vi "数据平滑.vi"(8 "Reference data in":cluster{"参考数值":dbl[], "参考数值时间戳":timestamp[]}, 10 "Para":T2 {"切换阈值" format="%#_6f"}, 11 "data in":cluster{"数值":dbl, "时间标识":timestamp}) -> (0 "Reference data out":cluster{"参考数值":dbl[], "参考数值时间戳":timestamp[]}, 3 "data out":T1)   [LabVIEW 2016, in "仿真数据.lvlib"]
uses:
  <vilib>/Analysis/NI_AALBase.lvlib
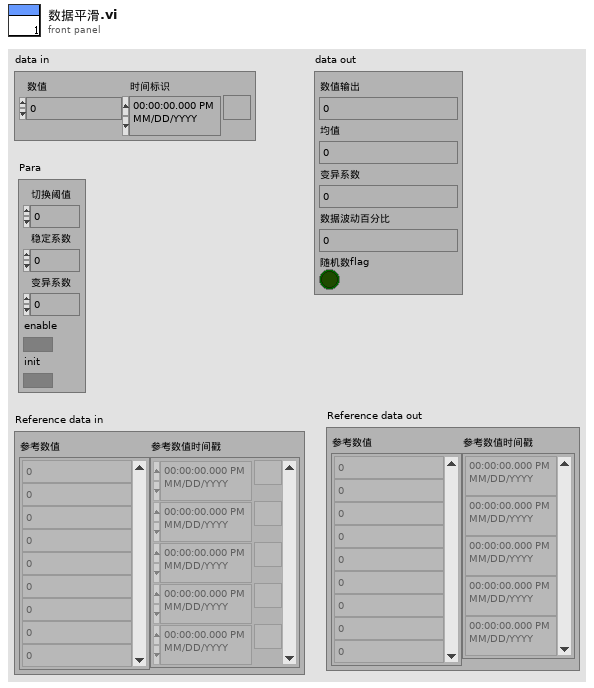
[diagram p1: front panel]
types:
  T1 = cluster{"数值输出":dbl, "均值":dbl, "变异系数":dbl, "数据波动百分比":dbl, "随机数flag":bool}
  T2 = cluster{"切换阈值":dbl, "稳定系数":dbl, "变异系数":dbl, "enable":bool, "init":bool}
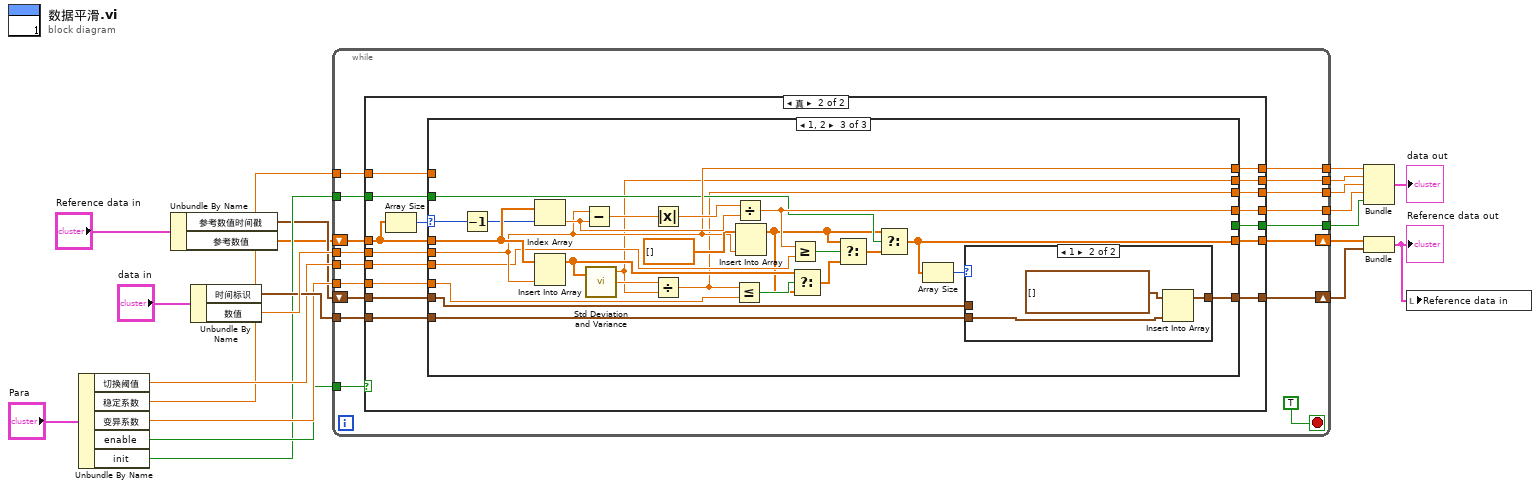
[diagram p0: block diagram]
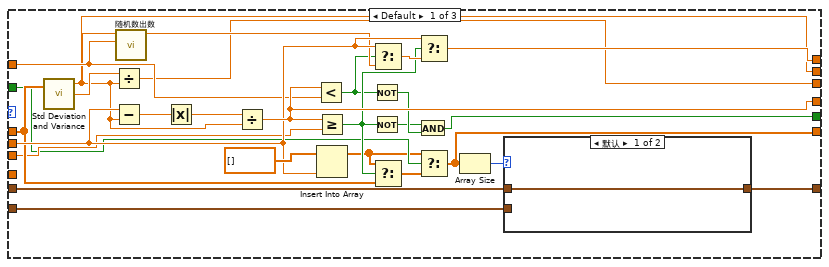
[diagram p3: hidden frame]
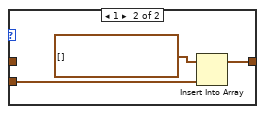
[diagram p4: hidden frame]
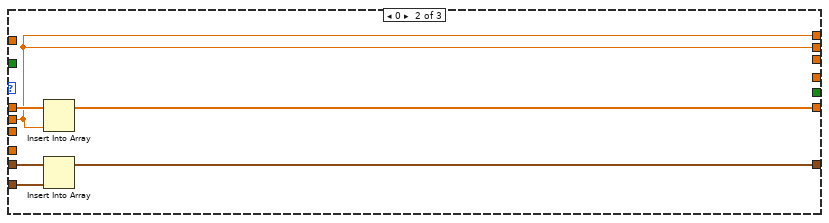
[diagram p5: hidden frame]
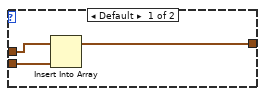
[diagram p6: hidden frame]
diagram:
  n1 = Unbundle By Name("Para") -> ("切换阈值"=w17:dbl, "稳定系数"=w16:dbl, "变异系数"=w15:dbl, "enable"=w14:bool, "init"=w13:bool)
  n2 = Unbundle By Name("Reference data in") -> ("参考数值时间戳"=w5:timestamp[], "参考数值"=w4:dbl[])
  n3 = Unbundle By Name("data in") -> ("时间标识"=w19:timestamp, "数值"=w20:dbl)
  n4 = while {
    tunnel: w20 -> [w36]
    shift-right: [w34] -> w3
    shift-left: w4 -> [w37]
    tunnel: [w35] -> w12
    tunnel: w16 -> [w33]
    tunnel: w17 -> [w32]
    tunnel: w15 -> [w31]
    tunnel: w14 -> [w30]
    tunnel: w19 -> [w29]
    shift-right: [w27] -> w2
    shift-left: w5 -> [w28]
    tunnel: w13 -> [w26]
    tunnel: [w25] -> w11
    tunnel: [w24] -> w10
    tunnel: [w23] -> w9
    tunnel: [w22] -> w8
    stop <- TRUE stop-if-true
    n5 = case shown="真" w30 {
      tunnel: w37 -> [_ w55]
      tunnel: w36 -> [w39 w54]
      tunnel: [w39 w53] -> w35
      tunnel: [_ w52] -> w34
      tunnel: w33 -> [_ w51]
      tunnel: w32 -> [_ w50]
      tunnel: w31 -> [_ w49]
      tunnel: [_ w48] -> w22
      tunnel: [_ w47] -> w23
      tunnel: w29 -> [_ w46]
      tunnel: w28 -> [_ w45]
      tunnel: [_ w44] -> w27
      tunnel: [_ w42] -> w24
      tunnel: [w39 w41] -> w25
      tunnel: w26 -> [_ w40]
      frame False {
      }
      frame True {
        n6 = Array Size(array=w55) -> (size(s)=w43:i32)
        n7 = case shown="1, 2" w43 {
          selector: w43 -> [_ _ w114]
          tunnel: w55 -> [w69 w92 w115]
          tunnel: [w60 w91 w96] -> w52
          tunnel: w54 -> [w77 w87 w110]
          tunnel: [w80 w87 w110] -> w53
          tunnel: [w78 _ w112] -> w47
          tunnel: [w70 _ _] -> w48
          tunnel: w51 -> [w68 _ _]
          tunnel: w50 -> [w67 _ w106]
          tunnel: w49 -> [_ _ w105]
          tunnel: w46 -> [w64 w90 w104]
          tunnel: w45 -> [w65 w89 w100]
          tunnel: [w63 w88 w99] -> w44
          tunnel: w40 -> [w62 _ w98]
          tunnel: [w57 _ w94] -> w42
          tunnel: [w56 w87 w93] -> w41
          frame Default {
            n8 = call <vilib>:"Std Deviation and Variance.vi"("X"=w69) -> ("mean"=w56:dbl, "standard deviation"=w58:dbl)  [unwired: 1 in, 1 out]
            n9 = Divide(x=w58, y=w56) -> (x/y=w57:dbl)
            n10 = Subtract(x=w77, y=w56) -> (x-y=w82:dbl)
            n11 = call "随机数出数.vi"("百分比"=w68, "输入"=w56) -> ("输出"=w76:dbl)  [unwired: 9 in]
            n12 = Absolute Value(x=w82) -> (abs(x)=w81:dbl)
            n13 = Divide(x=w81, y=w56) -> (x/y=w78:dbl)
            n14 = Less?(x=w78, y=w68) -> (x < y?=w73:bool)
            n15 = Greater Or Equal?(x=w78, y=w67) -> (x >= y?=w74:bool)
            n16 = Insert Into Array(array=dbl[] [], new element=w77) -> (w59:dbl[])  [unwired: 1 in]
            n17 = Not(x=w73) -> (.not. x?=w72:bool)
            n18 = Not(x=w74) -> (.not. x?=w71:bool)
            n19 = Select(t=w77, s=w73, f=w76) -> (s? t:f=w75:dbl)
            n20 = Select(t=w59, s=w74, f=w69) -> (s? t:f=w61:dbl[])
            n21 = And(x=w71, y=w72) -> (x .and. y?=w70:bool)
            n22 = Select(t=w77, s=w74, f=w75) -> (s? t:f=w80:dbl)
            n23 = Select(t=w59, s=w62, f=w61) -> (s? t:f=w60:dbl[])
            n24 = Array Size(array=w60) -> (size(s)=w66:i32)
            n25 = case shown="默认" w66 {
              tunnel: w64 -> [_ w85]
              tunnel: [w83 w84] -> w63
              tunnel: w65 -> [w83 _]
              frame Default {
              }
              frame 1 {
                n26 = Insert Into Array(array=timestamp[] [], new element=w85) -> (w84:timestamp[])  [unwired: 1 in]
              }
            }
          }
          frame 0 {
            n27 = Insert Into Array(array=w92, new element=w87) -> (w91:dbl[])  [unwired: 1 in]
            n28 = Insert Into Array(array=w89, new element=w90) -> (w88:timestamp[])  [unwired: 1 in]
          }
          frame 1, 2 {
            n29 = Decrement(x=w114) -> (x-1=w113:i32)
            n30 = Index Array(array=w115, index=w113) -> (element=w116:dbl)
            n31 = Insert Into Array(array=w115, new element=w110) -> (w108:dbl[])  [unwired: 1 in]
            n32 = Subtract(x=w110, y=w116) -> (x-y=w118:dbl)
            n33 = call <vilib>:"Std Deviation and Variance.vi"("X"=w108) -> ("mean"=w93:dbl, "standard deviation"=w109:dbl)  [unwired: 1 in, 1 out]
            n34 = Absolute Value(x=w118) -> (abs(x)=w117:dbl)
            n35 = Divide(x=w109, y=w93) -> (x/y=w94:dbl)
            n36 = Less Or Equal?(x=w94, y=w105) -> (x <= y?=w103:bool)
            n37 = Divide(x=w117, y=w116) -> (x/y=w112:dbl)
            n38 = Insert Into Array(array=dbl[] [], new element=w110) -> (w95:dbl[])  [unwired: 1 in]
            n39 = Greater Or Equal?(x=w112, y=w106) -> (x >= y?=w102:bool)
            n40 = Select(t=w108, s=w103, f=w95) -> (s? t:f=w107:dbl[])
            n41 = Select(t=w95, s=w102, f=w107) -> (s? t:f=w97:dbl[])
            n42 = Select(t=w95, s=w98, f=w97) -> (s? t:f=w96:dbl[])
            n43 = Array Size(array=w96) -> (size(s)=w101:i32)
            n44 = case shown="1" w101 {
              tunnel: w104 -> [w120 w123]
              tunnel: [w119 w122] -> w99
              tunnel: w100 -> [w121 _]
              frame Default {
                n45 = Insert Into Array(array=w121, new element=w120) -> (w119:timestamp[])  [unwired: 1 in]
              }
              frame 1 {
                n46 = Insert Into Array(array=timestamp[] [], new element=w123) -> (w122:timestamp[])  [unwired: 1 in]
              }
            }
          }
        }
      }
    }
  }
  n47 = Bundle("数值"=w12, "mean"=w11, w10, w9, w8) -> (→"data out":cluster{"数值":dbl, "mean":dbl, dbl, dbl, bool})  [unwired: 1 in]
  n48 = Bundle("参考数值"=w3, "参考数值时间戳"=w2) -> (w1:cluster{"参考数值":dbl[], "参考数值时间戳":timestamp[]})  [unwired: 1 in]
  "Reference data out" <- w1
  n49 = local write "Reference data in"(w1) -> ()
